vi "LaserMarked_SetPanel.vi"(11 "SetPanelRef":refnum<vi>) -> ()   [LabVIEW 2019]
uses:
  <vilib>/Utility/miscctls.llb/LVPointTypeDef.ctl
  <vilib>/Utility/miscctls.llb/LVPositionTypeDef.ctl
panel:
  in  "$S2 Dect No":i32 caption="S2探針使用次數" min=0 step=1
  in  "$Fire No Set":i32 caption="焊接次數設定" min=0 step=1
  in  "$S11_PreventionChk 1":i32 caption="S11 雷射測高檢知氣缸" min=0 step=1
  in  "$Laser Dect No":i32 caption="雷射測高次數" min=0 step=1
  in  "$Fire Connect No":i32 caption="熱熔次數設定" min=0 step=1
  in  "$S4 Dect No":i32 caption="S4探針使用次數" min=0 step=1
  in  "$S3 Dect No":i32 caption="S3探針使用次數" min=0 step=1
  in  "$VISA resource name 2":refnum<visa-resource-name> caption="IO板端口"
  in  "$Laser Tool Y":dbl caption="雷射測距Y距離(mm)" min=0.0 step=0.001 format="%#_4g"
  in  "$Laser Tool X":dbl caption="雷射測距X距離(mm)" min=0.0 step=0.001 format="%#_4g"
  in  "$MK ToolY":dbl caption="相機Y距離(mm)" min=0.0 step=0.001 format="%#_4g"
  in  "$MK ToolX":dbl caption="相機X距離(mm)" min=0.0 step=0.001 format="%#_4g"
  in  "$VISA resource name":refnum<visa-resource-name>
  in  "$Standar VNum_":string caption="標準電壓"
  in  "$Bin V DiffNum_":dbl caption="電壓差(V)" min=0.0 step=0.001 format="%#_4g"
  in  "$VType":enum16{"無條件捨去", "四捨五入"}(ring) caption="電壓選取方式"
  in  "$Ring":u16(ring) caption="Ring" items=["A", "V", "C"]
  in  "Tab Control":enum32{"S1~S4", "S5~S10", "S11~S13"}(tab)
  in  "$S1_PreventionChk 1":i32 caption="S1 檢平確認氣缸" min=0 step=1
  in  "$S1_PreventionChk 2":i32 caption="S1 電路板檢平On次數" min=0 step=1
  in  "$S1_PreventionChk 3":i32 caption="S1 電池檢平On次數" min=0 step=1
  in  "$S1_PreventionChk 4":i32 caption="S1 盒蓋檢平On次數" min=0 step=1
  in  "$S2_PreventionChk 1":i32 caption="S2 電流量測探針使用次數" min=0 step=1
  in  "$S2_PreventionChk 2":i32 caption="S2 電流量測氣缸" min=0 step=1
  in  "$S3_PreventionChk 1":i32 caption="S3程式燒入探針使用次數" min=0 step=1
  in  "$S3_PreventionChk 2":i32 caption="S3 程式燒入氣缸" min=0 step=1
  in  "$S4_PreventionChk 1":i32 caption="S4電壓量測探針使用次數" min=0 step=1
  in  "$S4_PreventionChk 2":i32 caption="S4電源3V探針使用次數" min=0 step=1
  in  "$S4_PreventionChk 3":i32 caption="S4 隔離箱上蓋氣缸" min=0 step=1
  in  "$S4_PreventionChk 4":i32 caption="S4 隔離箱下蓋氣缸" min=0 step=1
  in  "$S4_PreventionChk 5":i32 caption="S4 電池電壓量測固定氣缸" min=0 step=1
  in  "$S4_PreventionChk 6":i32 caption="S4 電池電壓量測氣缸" min=0 step=1
  in  "$S4_PreventionChk 7":i32 caption="S4 電路板檢測氣缸" min=0 step=1
  in  "$BypassModbus":bool caption="BypassModbusChk"
  in  "$AlarmCycleNo_S2":i16 caption="AlarmCycleNo_S2" min=0 step=1
  in  "$AlarmCycleNo_S3":i16 caption="AlarmCycleNo_S3" min=0 step=1
  in  "$AlarmCycleNo_S4":i16 caption="AlarmCycleNo_S4" min=0 step=1
  in  "$AlarmCycleNo_S11":i16 caption="AlarmCycleNo_S11" min=0 step=1
  in  "$S5_PreventionChk 1":i32 caption="S5 電路板取料升降氣缸" min=0 step=1
  in  "$S5_PreventionChk 3":i32 caption="S5 真空 吸取" min=0 step=1
  in  "$S5_PreventionChk 2":i32 caption="S5 電路板取料橫移氣缸" min=0 step=1
  in  "$S5_PreventionChk 4":i32 caption="S5 真空 解除" min=0 step=1
  in  "$S7_PreventionChk 1":i32 caption="S7 焊接料件固定氣缸" min=0 step=1
  in  "$S7_PreventionChk 2":i32 caption="S7 焊接機清錫馬達" min=0 step=1
  in  "$S10_PreventionChk 1":i32 caption="S10 料件翻轉區升降氣缸" min=0 step=1
  in  "$S10_PreventionChk 2":i32 caption="S10 料件翻轉區伸出氣缸" min=0 step=1
  in  "$S10_PreventionChk 3":i32 caption="S10 料件翻轉區旋轉氣缸" min=0 step=1
  in  "$S10_PreventionChk 4":i32 caption="S10 料件翻轉區夾取氣缸" min=0 step=1
  in  "$S10_PreventionChk 5":i32 caption="S10 料件橫移氣缸" min=0 step=1
  in  "$S10_PreventionChk 6":i32 caption="S10 料件吸取升降氣缸" min=0 step=1
  in  "$S10_PreventionChk 7":i32 caption="S10 料件放料升降氣缸" min=0 step=1
  in  "$S10_PreventionChk 8":i32 caption="S10 真空 吸取" min=0 step=1
  in  "$S10_PreventionChk 9":i32 caption="S10 真空 解除" min=0 step=1
  in  "$S12_PreventionChk 1":i32 caption="S12 熱熔升降氣缸" min=0 step=1
  in  "$S12_PreventionChk 2":i32 caption="S12 預熱升降氣缸" min=0 step=1
  in  "$S12_PreventionChk 3":i32 caption="S12 離子槍風速調控" min=0 step=1
  in  "$S13_PreventionChk 1":i32 caption="S13 真空 吸取" min=0 step=1
  in  "$S13_PreventionChk 2":i32 caption="S13 真空 解除" min=0 step=1
  in  "$S13_PreventionChk 3":i32 caption="S13 NG蓋取料夾爪" min=0 step=1
  in  "$S13_PreventionChk 4":i32 caption="S13 NG蓋取料升降" min=0 step=1
  in  "$S13_PreventionChk 5":i32 caption="S13 NG電池取料升降" min=0 step=1
  in  "$S13_PreventionChk 6":i32 caption="S13 NG電路板取料升降" min=0 step=1
  in  "$S13_PreventionChk 7":i32 caption="S13 NG橫移氣缸" min=0 step=1
  in  "$S13_PreventionChk 8":i32 caption="S13 NG橫移氣缸" min=0 step=1
  in  "$S12_PreventionChk 4":i32 caption="S12 熱熔次數" min=0 step=1
  in  "$S11_PreventionChk 1":i32 caption="S11 雷射檢測次數" min=0 step=1
  in  "$S7_PreventionChk 3":i32 caption="S7 焊接啟動次數" min=0 step=1
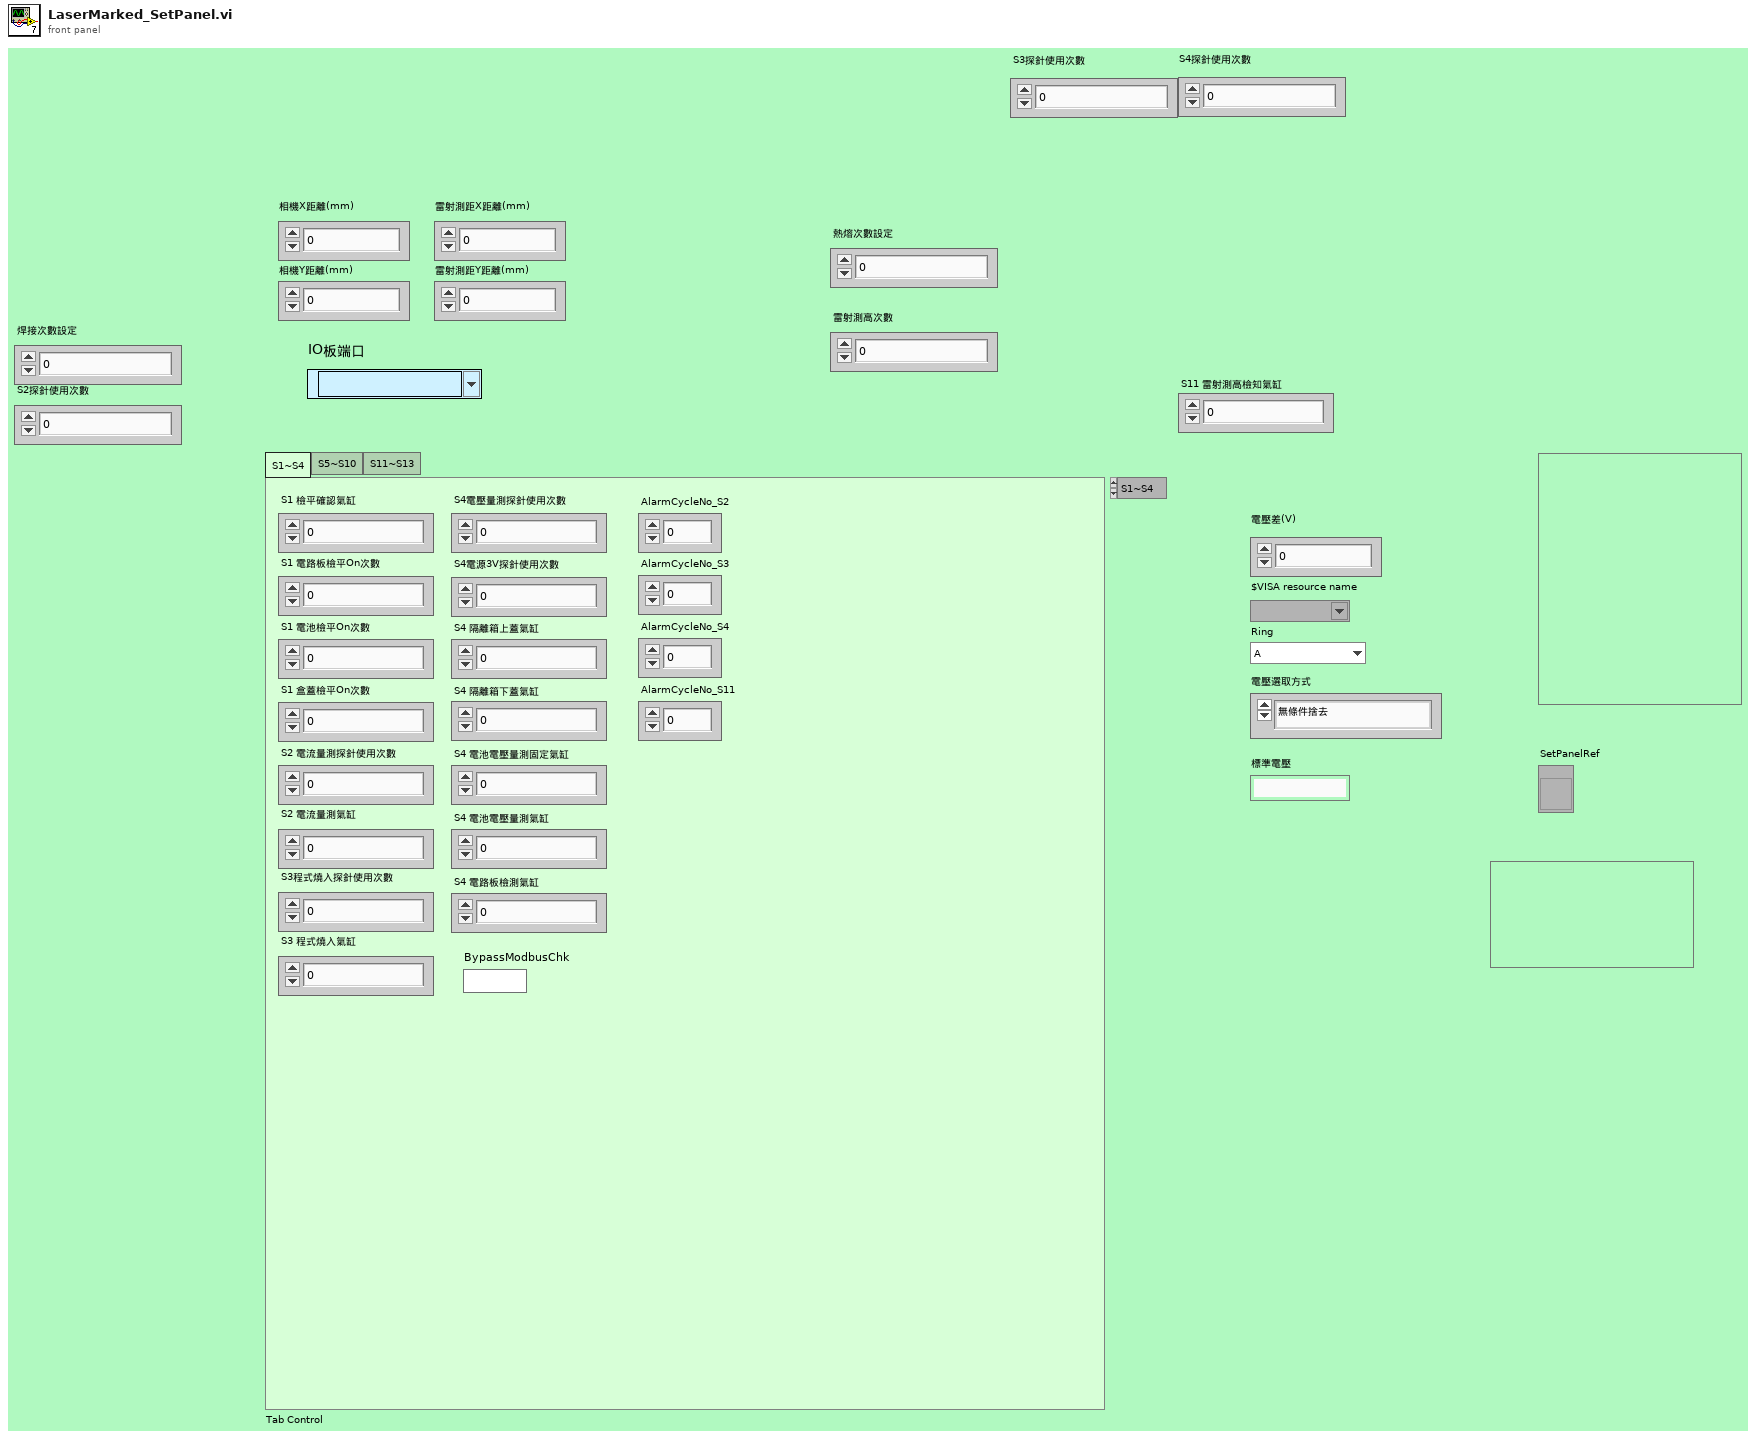
[diagram p1: front panel]
types:
  T1 = typedef "LVPositionTypeDef.ctl" = cluster{"Left":i32, "Top":i32}
  T2 = typedef "LVPointTypeDef.ctl" = cluster{"Horizontal":i16, "Vertical":i16}
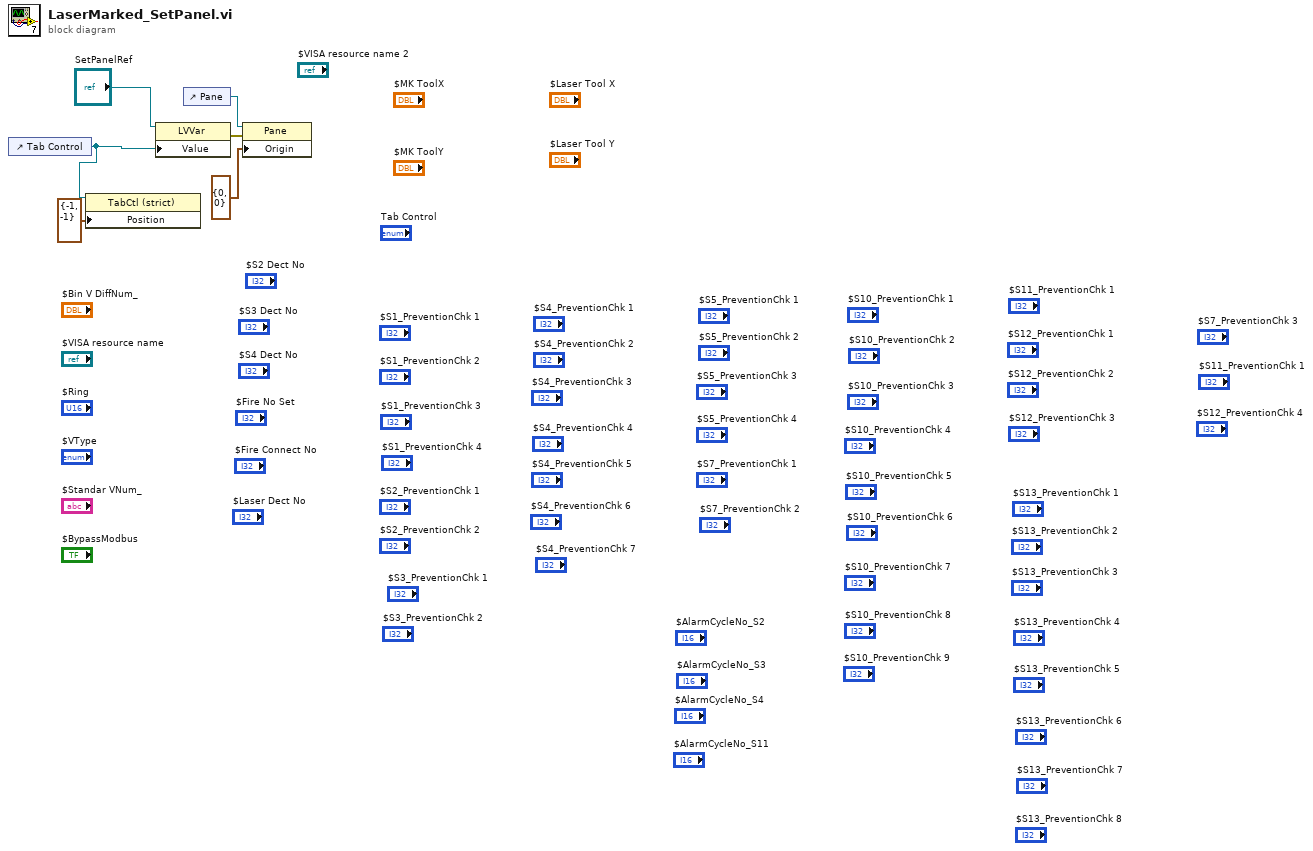
[diagram p0: block diagram]
diagram:
  n1 = control-ref of="Tab Control"() -> (w2:refnum<vi>)
  n2 = property class="TabCtl (strict)"(reference=w2, "Position"=T1 {"Left"=-1, "Top"=-1}) -> ()  [unwired: 1 in, 2 out]
  n3 = property class="LVVar"(reference="SetPanelRef", "Value"=w2) -> (error out=w3:errorcluster)  [unwired: 1 in, 1 out]
  n4 = control-ref of="Pane"() -> (w4:refnum<vi>)
  n5 = property class="Pane"(reference=w4, error in=w3, "Origin"=T2 {"Horizontal"=0, "Vertical"=0}) -> ()  [unwired: 2 out]
